vi "Open port.vi"(8 "error in (no error)":errorcluster, 11 "Serial Base in":refnum<class "Serial Base.lvclass">) -> (0 "error out":errorcluster, 3 "Serial Base out":refnum<class "Serial Base.lvclass">)   [LabVIEW 2022 SP3, in "Serial Base.lvclass"]
uses:
  Serial Base.lvclass
  Serial Base.lvclass/Serial Base.ctl
  <vilib>/Instr/_visa.llb/VISA Configure Serial Port (Instr).vi
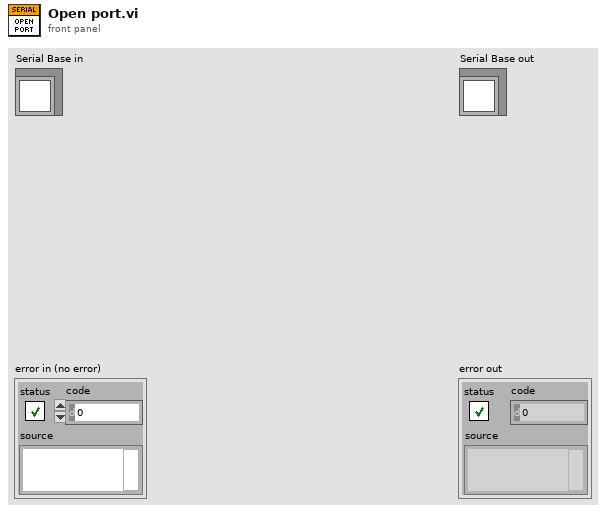
[diagram p1: front panel]
types:
  T1 = typedef "Serial Base.lvclass/Object Argument--cluster.ctl" = cluster{"Com Port":refnum<visa-resource-name>, "baud rate":u32, "data bits":u16, "Termination Char":T2, "parity":enum16{"None", "Odd", "Even", "Mark", "Space"}, "stop bits":u16, "flow control ":u16, "timeout ":u32}
  T2 = typedef "Serial Base.lvclass/Termination Character--enum.ctl" = enum16{"none", "\\r\\n", "\\r", "\\n"}
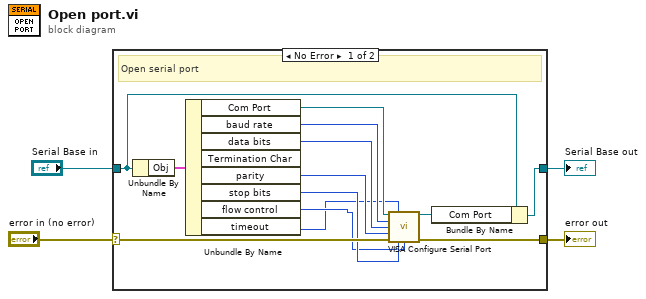
[diagram p0: block diagram]
diagram:
  n1 = case shown="No Error" "error in (no error)" {
    selector: "error in (no error)" -> [w15 w19]
    tunnel: [w9 w19] -> w3
    tunnel: [w16 w18] -> w1
    tunnel: "Serial Base in" -> [w17 w18]
    frame No Error {
      # "Open serial port"
      n2 = Unbundle By Name(w17) -> ("Obj"=w14:T1)
      n3 = Unbundle By Name(w14) -> ("Com Port"=w13:refnum<visa-resource-name>, "baud rate"=w12:u32, "data bits"=w11:u16, "parity"=w10:enum16{"None", "Odd", "Even", "Mark", "Space"}, "stop bits"=w8:u16, "flow control"=w7:u16, "timeout"=w5:u32)  [unwired: 1 out]
      n4 = call-poly "VISA Configure Serial Port"("VISA resource name"=w13, "timeout (10sec)"=w5, "baud rate (9600)"=w12, "data bits (8)"=w11, "parity (0:none)"=w10, "error in (no error)"=w15, "stop bits (10: 1 bit)"=w8, "flow control (0:none)"=w7) -> ("VISA resource name out"=w6:refnum<visa-resource-name>, "error out"=w9:errorcluster)  [unwired: 6 in]
      n5 = Bundle By Name(cluster=w17, "Com Port"=w6) -> (w16:refnum<class "Serial Base.lvclass">)
    }
    frame Error {
    }
  }
  "error out" <- w3
  "Serial Base out" <- w1
